vi "Inspect State Exec 0.vi"(8 "error in (no error)":errorcluster, 11 "Image Src":T1) -> (0 "error out":errorcluster, 3 "Image Out":T1)   [LabVIEW 2019]
uses:
  <vilib>/vision/Image Controls.llb/IMAQ Image.ctl
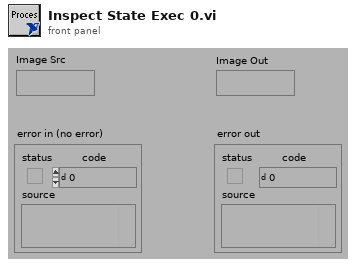
[diagram p1: front panel]
types:
  T1 = typedef "IMAQ Image.ctl" = refnum<image>
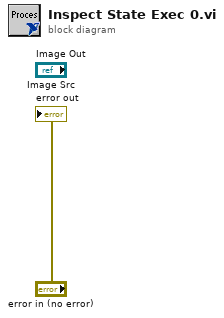
[diagram p0: block diagram]
diagram:
  "Image Out" <- "Image Src"
  "error out" <- "error in (no error)"
